vi "Lift Controller.vi"(8 "error in":errorcluster) -> ()   [LabVIEW 2017]
doc: "This VI executes continuously carrying out the current operation and responding to updates or new operations. It will often contain the timing or control code that is difficult to place directly in TeleOp. This VI generally opens all sensors and motors and isolates the rest of the robot code from knowing how the operations are carried out."
uses:
  Lift Operations.ctl
  Lift Setpoints.ctl
  <vilib>/Rock Robotics/WPI/SafetyOutput/WPI_SafetyOutputConfigMenu.ctl
  <vilib>/Rock Robotics/Network Tables/NT Write Boolean.vi
  <vilib>/Rock Robotics/WPI/Framework/Completion Status.ctl
panel:
  in  "Slide 2":dbl(slide) scale=-1.0..1.0
  in  "Slide":dbl(slide) scale=-1.0..1.0
  in  "Interactive Values":T1
  out "Current\nCmd":string
  in  "Buttons":cluster{"Execute Cmd":bool, "Abort Cmd":bool}
  out "Command Timing":cluster{"Start Time (ms)":u32, "Iterations":i32}
  out "Status":T3
  # "Tip: It may be helpful to observe inputs and sensor values.\nYou may also want to display tuning or debugging controls."
  # "Interactive Command: You may fill in the settings for a command\nand schedule it with the Execute button. You can observe and abort\nany command while fine tuning the code for the controller."
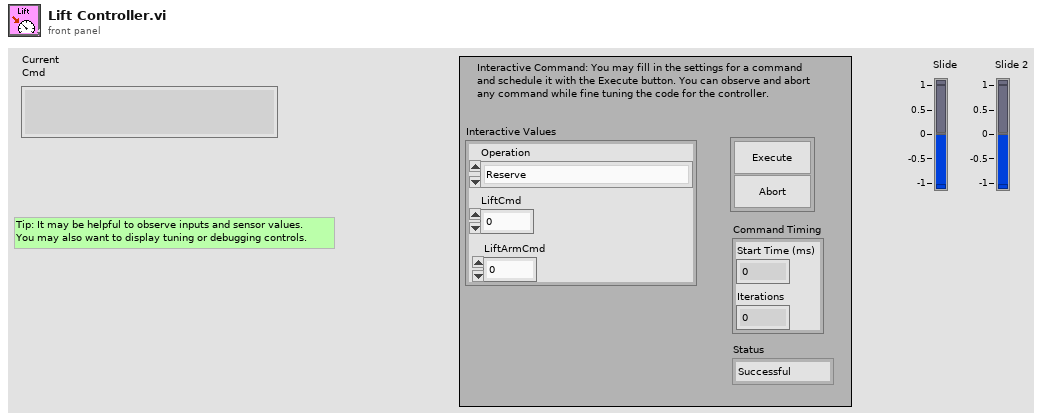
[diagram p1: front panel]
types:
  T1 = typedef "Lift Setpoints.ctl" = cluster{"Operation":T2, "LiftCmd":dbl, "LiftArmCmd":dbl}
  T2 = typedef "Lift Operations.ctl" = enum16{"Reserve", "Read Current", "Immediate"}
  T3 = typedef "Completion Status.ctl" = enum16{"Successful", "Aborted", "Incomplete"}
  T4 = typedef "WPI_SafetyOutputConfigMenu.ctl" = enum16{"Enable", "Disable"}
  T5 = typedef "WPI_MotorControlDeviceRef.ctl" = cluster{"DeviceStatus":errorcluster, "Type":T6, "PWM":cluster{"PWM Channel":T7, "DeadBand":T8}, "CAN":cluster{"Device Number":u8, "SetOutput VI Ref":variant, "GetOutput VI Ref":variant, "Enable VI Ref":variant, "Disable VI Ref":variant, "Data":variant}, "Invert":bool, "DIO PWM":cluster{"PWM \"Enable\" Channel":T7, "DIOChannel":T9, "PWM Rate":dbl}}
  T6 = typedef "WPI_MotorControlType.ctl" = enum16{"PWM", "CAN", "DIO PWM"}
  T7 = typedef "FPGA_DIOPWMChannel.ctl" = enum8{"PWM 0", "PWM 1", "PWM 2", "PWM 3", "PWM 4", "PWM 5", "PWM 6", "PWM 7", "PWM 8", "PWM 9", "PWM MXP 0", "PWM MXP 1", "PWM MXP 2", "PWM MXP 3", "PWM MXP 4", "PWM MXP 5", "PWM MXP 6", "PWM MXP 7", "PWM MXP 8", "PWM MXP 9", "Invalid"}
  T8 = typedef "WPI_PWMDeadband.ctl" = cluster{"Name":string, "maxPositivePwm":i32, "minPositivePwm":i32, "centerPwm":i32, "maxNegativePwm":i32, "minNegativePwm":i32, "angularRange":u16}
  T9 = typedef "FPGA_DIOChannel.ctl" = enum8{"DIO 0", "DIO 1", "DIO 2", "DIO 3", "DIO 4", "DIO 5", "DIO 6", "DIO 7", "DIO 8", "DIO 9", "DIO MXP 0", "DIO MXP 1", "DIO MXP 2", "DIO MXP 3", "DIO MXP 4", "DIO MXP 5", "DIO MXP 6", "DIO MXP 7", "DIO MXP 8", "DIO MXP 9", "DIO MXP 10", "DIO MXP 11", "DIO MXP 12", "DIO MXP 13", "DIO MXP 14", "DIO MXP 15", "SPI Port CS1", "SPI Port CS2", "SPI Port CS3", "SPI Port MISO", "SPI Port MOSI", "Invalid"}
  T10 = typedef "Command Status Info.ctl" = cluster{"Name":string, "Status":T3, "notifier out":T11}
  T11 = typedef "Completion Notifier.ctl" = refnum<notifier>
  T12 = cluster{"Current Command":T1, "Command Timing":cluster{"Start Time (ms)":u32, "Iterations":i32}, "Command Arguments":cluster{"Command Info":T10, "Description":string, "Default Command":T1, "queue out":refnum<queue>, "Subsystem Name":string}}
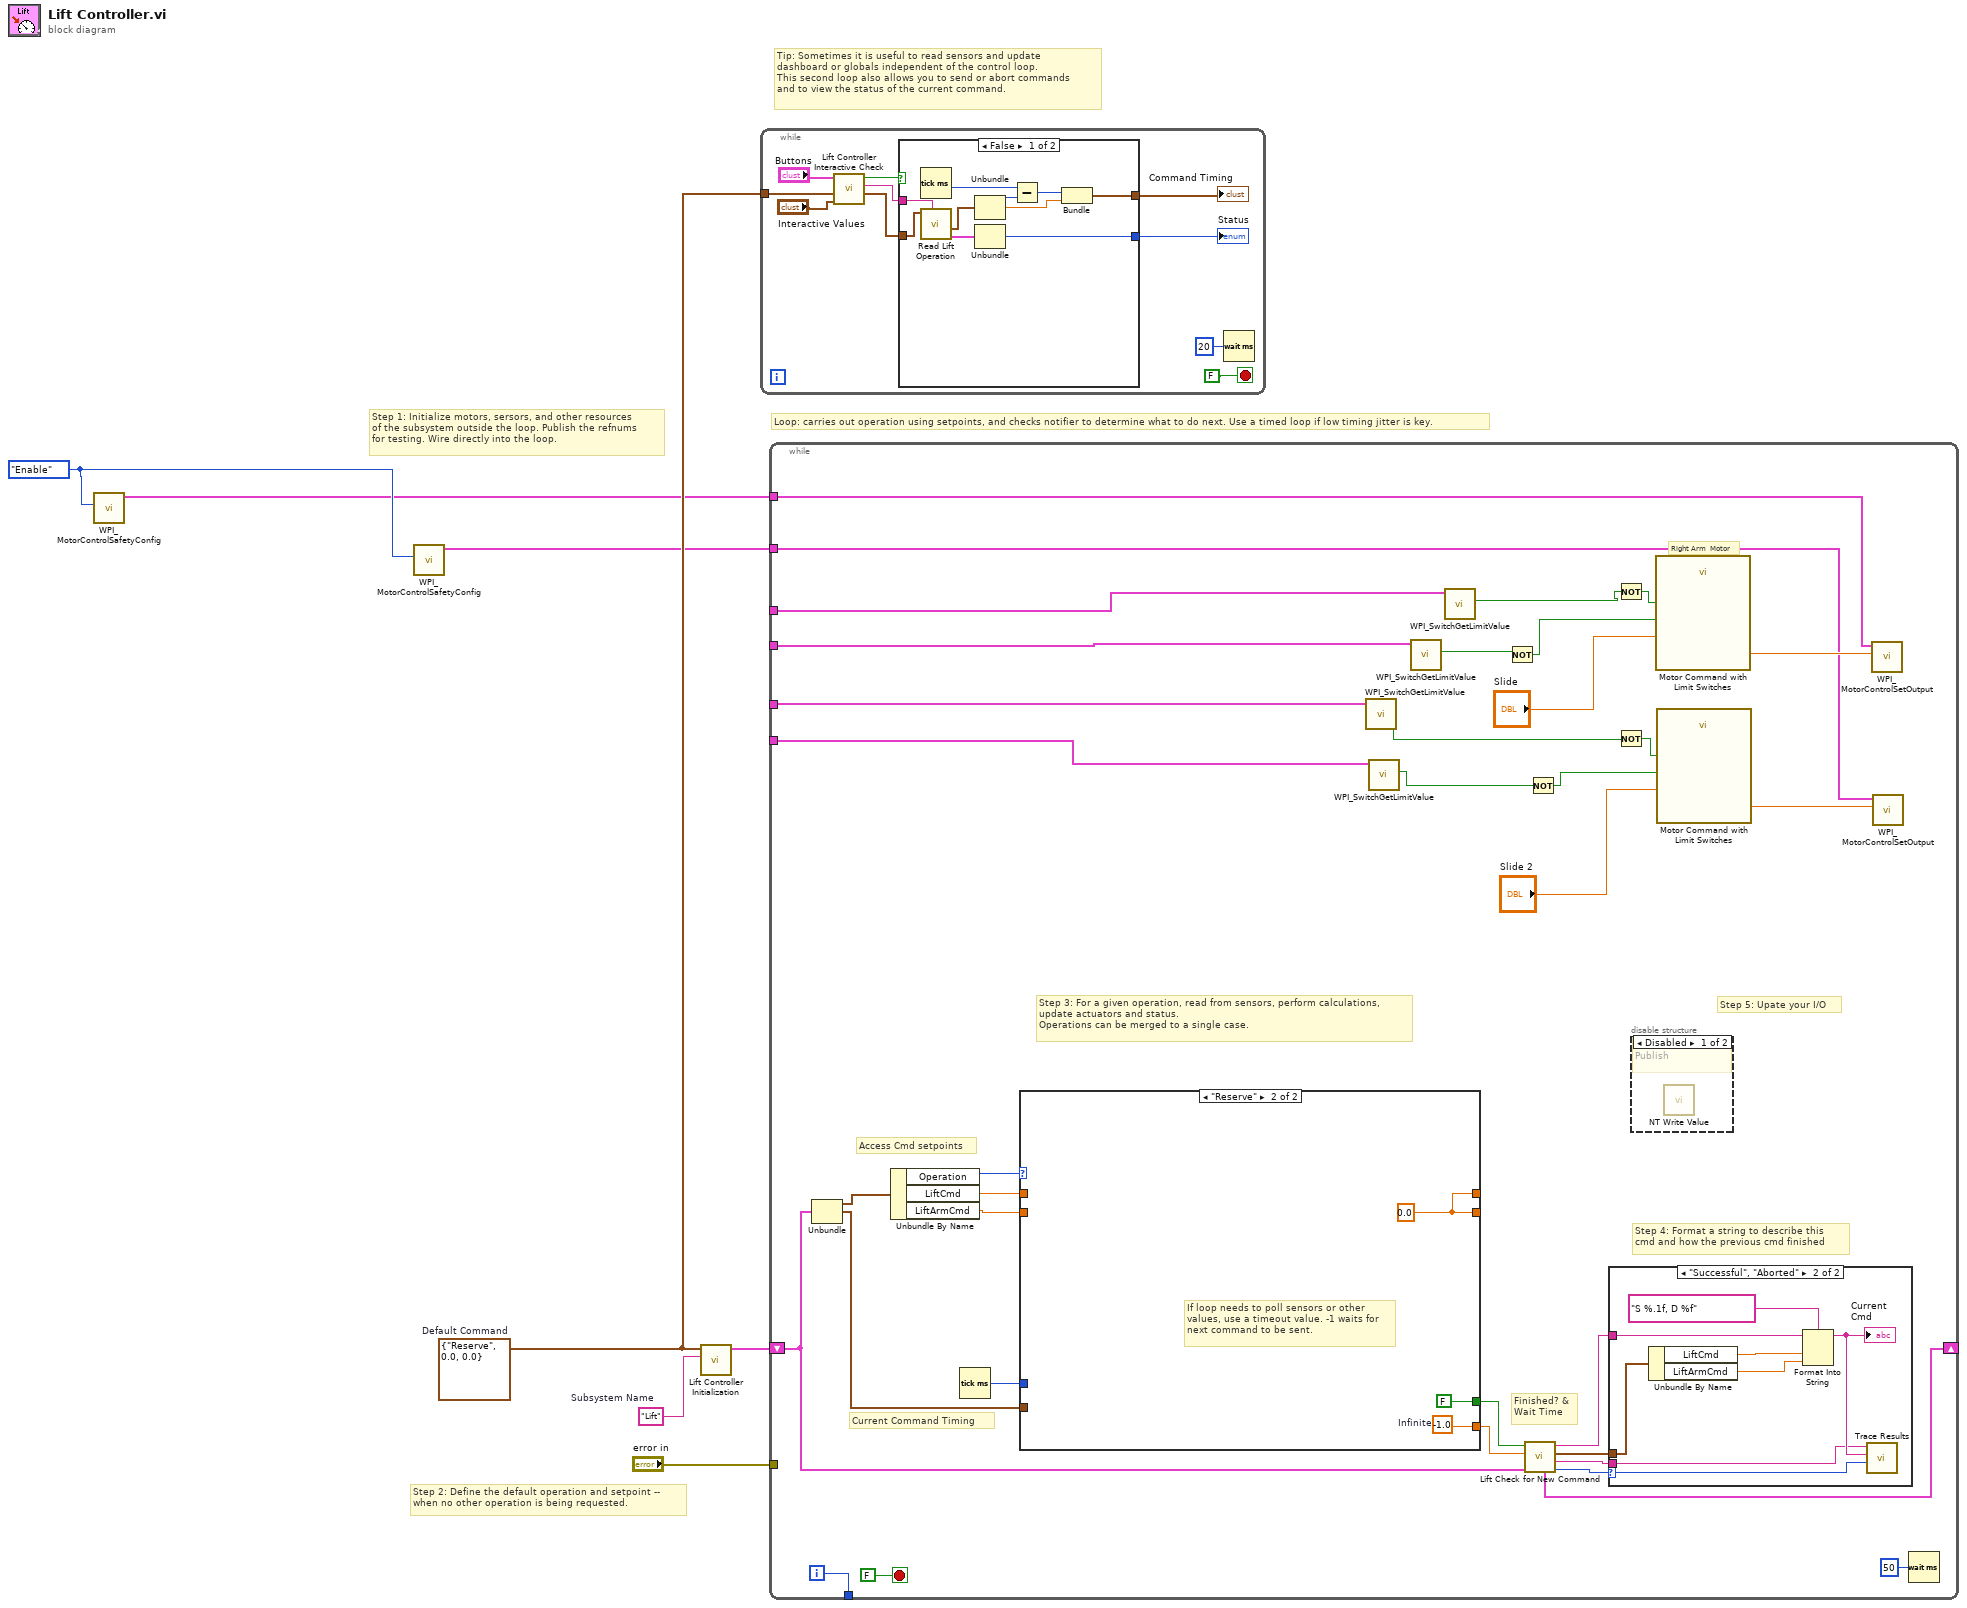
[diagram p0: block diagram]
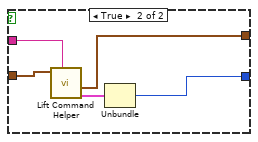
[diagram p2: hidden frame]
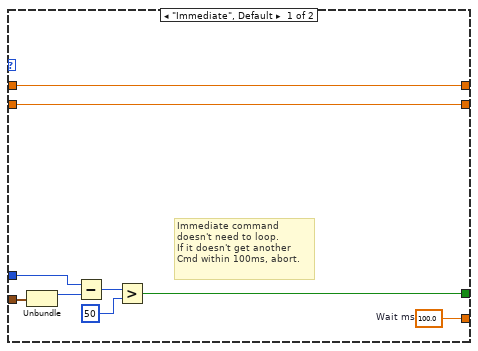
[diagram p5: hidden frame]
diagram:
  w7 = WPI_SafetyOutputConfigMenu."Enable" ("mode")
  w8 = T1 {"Operation"=enum."Reserve", "LiftCmd"=0.0, "LiftArmCmd"=0.0}  # Default Command
  w9 = "Lift"  # Subsystem Name
  # "Tip: Sometimes it is useful to read sensors and update\ndashboard or globals independent of the control loop.\nThis second loop also allows you to send or abort commands\nand to view the status of the current command."
  # "Step 2: Define the default operation and setpoint --\nwhen no other operation is being requested."
  # "Step 1: Initialize motors, sersors, and other resources\nof the subsystem outside the loop. Publish the refnums\nfor testing. Wire directly into the loop."
  # "Loop: carries out operation using setpoints, and checks notifier to determine what to do next. Use a timed loop if low timing jitter is key."
  n1 = call <vilib>:"WPI_MotorControlSafetyConfig.vi"("mode"=w7) -> ("MotorControlDevRef"=w6:T5)  [unwired: 9 in, 1 out]
  n2 = call <vilib>:"WPI_MotorControlSafetyConfig.vi"("mode"=w7) -> ("MotorControlDevRef"=w5:T5)  [unwired: 9 in, 1 out]
  n3 = call "Lift Controller Initialization.vi"("Subsystem Name"=w9, "Default Command"=w8) -> ("Current Command"=w10:T12)  [unwired: 9 in]
  n4 = while {
    tunnel: w8 -> [w18]
    stop <- FALSE stop-if-true
    n5 = call "Lift Controller Interactive Check.vi"("Interactive Command in"="Interactive Values", "Default Command"=w18, "Buttons"="Buttons") -> ("Interactive Command out"=w15:T1, "Trace String"=w16:string, "Schedule"=w17:bool)  [unwired: 6 in]
    n6 = case shown="False" w17 {
      tunnel: [w31 w36] -> w14
      tunnel: w15 -> [w22 w34]
      tunnel: [w27 w32] -> w13
      tunnel: w16 -> [w23 w35]
      frame False {
        n7 = Tick Count (ms)() -> (millisecond timer value=w26:u32)
        n8 = call "Read Lift Operation.vi"("Description"=w23, "SubSystem Data 2"=w22) -> ("Command Info"=w24:T10, "SubSystem Data"=w25:T1)  [unwired: 7 in, 1 out]
        n9 = Unbundle(w25) -> ("Operation"=w30:T2, "LiftCmd"=w28:dbl)  [unwired: 1 out]
        n10 = Unbundle(w24) -> ("Status"=w31:T3)  [unwired: 2 out]
        n11 = Subtract(x=w26, y=w30) -> (x-y=w29:u32)
        n12 = Bundle(w29, "LiftCmd"=w28) -> (w27:cluster{u32, "LiftCmd":dbl})  [unwired: 1 in]
      }
      frame True {
        n13 = call "Lift Command Helper.vi"("Description"=w35, "SubSystem Data"=w34) -> ("Command Info Out"=w33:T10, "Command Timing"=w32:cluster{"Start Time (ms)":u32, "Iterations":i32})  [unwired: 7 in, 1 out]
        n14 = Unbundle(w33) -> ("Status"=w36:T3)  [unwired: 2 out]
      }
    }
    "Status" <- w14
    "Command Timing" <- w13
    n15 = Wait (ms)(milliseconds to wait=u32 20) -> ()  [unwired: 1 out]
  }
  n16 = while {
    shift-right: [w64] -> _
    shift-left: w10 -> [w57]
    tunnel: [w70] -> _
    tunnel: "error in" -> [_]
    tunnel: w6 -> [w54]
    tunnel: w5 -> [w48]
    tunnel: [w52] -> w4
    tunnel: [w53] -> w3
    tunnel: [w50] -> w2
    tunnel: [w49] -> w1
    i -> [w70]
    stop <- FALSE stop-if-true
    # "Right Arm  Motor"
    # "Step 5: Upate your I/O"
    # "Step 4: Format a string to describe this\ncmd and how the previous cmd finished"
    # "Current Command Timing"
    # "Access Cmd setpoints"
    # "Finished? &\nWait Time"
    # "Step 3: For a given operation, read from sensors, perform calculations,\nupdate actuators and status.\nOperations can be merged to a single case."
    n17 = Unbundle(w57) -> ("Current Command"=w69:T1, "Command Timing"=w66:cluster{"Start Time (ms)":u32, "Iterations":i32})  [unwired: 1 out]
    n18 = Unbundle By Name(w69) -> ("Operation"=w68:T2, "LiftCmd"=w39:dbl, "LiftArmCmd"=w65:dbl)
    n19 = Tick Count (ms)() -> (millisecond timer value=w67:u32)
    n20 = case shown="\"Reserve\"" w68 {
      tunnel: [w88 w91] -> w62
      tunnel: [w82 FALSE ("ignore previous (F)")] -> w63
      tunnel: w66 -> [w84 _]
      tunnel: w67 -> [w83 _]
      tunnel: w65 -> [w81 _]
      tunnel: [w81 w89] -> _
      tunnel: w39 -> [w80 _]
      tunnel: [w80 w89] -> _
      frame "Immediate", Default {
        w88 = 100.0  # Wait ms
        # "Immediate command\ndoesn't need to loop.\nIf it doesn't get another\nCmd within 100ms, abort."
        n21 = Unbundle(w84) -> ("Start Time (ms)"=w87:u32)  [unwired: 1 out]
        n22 = Subtract(x=w83, y=w87) -> (x-y=w86:u32)
        n23 = Greater?(x=w86, y=u8 50 ("Left Motor")) -> (0:w82:bool)
      }
      frame "Reserve" {
        w89 = 0.0 ("LiftCmd")
        w91 = -1.0  # Infinite
        # "If loop needs to poll sensors or other\nvalues, use a timeout value. -1 waits for\nnext command to be sent."
      }
    }
    n24 = call <vilib>:"WPI_SwitchGetLimitValue.vi"("SwitchDevRef"=w50) -> ("Switch Pressed"=w45:bool)  [unwired: 8 in, 2 out]
    n25 = call <vilib>:"WPI_SwitchGetLimitValue.vi"("SwitchDevRef"=w49) -> ("Switch Pressed"=w47:bool)  [unwired: 8 in, 2 out]
    n26 = call <vilib>:"WPI_SwitchGetLimitValue.vi"("SwitchDevRef"=w53) -> ("Switch Pressed"=w43:bool)  [unwired: 8 in, 2 out]
    n27 = call <vilib>:"WPI_SwitchGetLimitValue.vi"("SwitchDevRef"=w52) -> ("Switch Pressed"=w41:bool)  [unwired: 8 in, 2 out]
    n28 = Not(x=w43) -> (.not. x?=w42:bool)
    n29 = call "Lift Check for New Command.vi"("Current Command"=w57, "Wait time (ms)"=w62, "Finished?"=w63) -> ("Completion"=w58:T3, "Subsystem Name"=w59:string, "Current Command"=w60:T1, "Initial Trace String"=w61:string, "NextCommand"=w64:T12)  [unwired: 4 in]
    n30 = Not(x=w47) -> (.not. x?=w46:bool)
    n31 = case shown="\"Successful\", \"Aborted\"" w58 {
      selector: w58 -> [_ w79]
      tunnel: w61 -> [_ w75]
      tunnel: w60 -> [_ w76]
      tunnel: w59 -> [_ w72]
      frame "Incomplete", Default {
        # "Continuing current command"
      }
      frame "Successful", "Aborted" {
        # "Report and setup for next command"
        n32 = Unbundle By Name(w76) -> ("LiftCmd"=w78:dbl, "LiftArmCmd"=w73:dbl)
        n33 = Format Into String(format string="S %.1f, D %f", initial string=w75, w78, w73) -> (resulting string=w74:string)  [unwired: 1 in, 1 out]
        "Current\nCmd" <- w74
        n34 = call <vilib>:"Trace Results.vi"("Status of previous command"=w79, "Description"=w74, "Subsystem"=w72) -> ()  [unwired: 9 in]
      }
    }
    n35 = Not(x=w41) -> (.not. x?=w40:bool)
    n36 = Not(x=w45) -> (.not. x?=w44:bool)
    n37 = disable-structure shown="Disabled" {
      frame Disabled {
        # "Publish"
        n38 = call-poly <vilib>:"NT Write Value.vi"() -> ()  [unwired: 11 in, 1 out]
      }
      frame Enabled {
      }
    }
    n39 = call "Motor Command with Limit Switches.vi"("LowLimitSwitch"=w42, "MotorCommandIn"="Slide", "HighLimitSwitch"=w40) -> (0:w55:dbl)
    n40 = call "Motor Command with Limit Switches.vi"("LowLimitSwitch"=w46, "MotorCommandIn"="Slide 2", "HighLimitSwitch"=w44) -> (0:w51:dbl)
    n41 = call <vilib>:"WPI_MotorControlSetOutput.vi"("Output"=w55, "MotorControlDevRef"=w54) -> ()  [unwired: 7 in, 3 out]
    n42 = call <vilib>:"WPI_MotorControlSetOutput.vi"("Output"=w51, "MotorControlDevRef"=w48) -> ()  [unwired: 7 in, 3 out]
    n43 = Wait (ms)(milliseconds to wait=u32 50) -> ()  [unwired: 1 out]
  }
